vi "from string version 1-0-0.vi"(8 "error in (no error)":errorcluster, 10 "Data String":string, 11 "DAQmx Watchdog configuration in":refnum<class "DAQmx Watchdog configuration.lvclass">) -> (0 "error out":errorcluster, 3 "DAQmx Watchdog configuration out":refnum<class "DAQmx Watchdog configuration.lvclass">)   [LabVIEW 2014, in "DAQmx Watchdog configuration.lvclass"]
uses:
  DAQmx Watchdog configuration.lvclass
  DAQmx Watchdog configuration.lvclass/DAQmx Watchdog configuration.ctl
  <vilib>/NI/Configuration Framework/serializable configuration/NISE_CEF_serializable configuration.lvclass
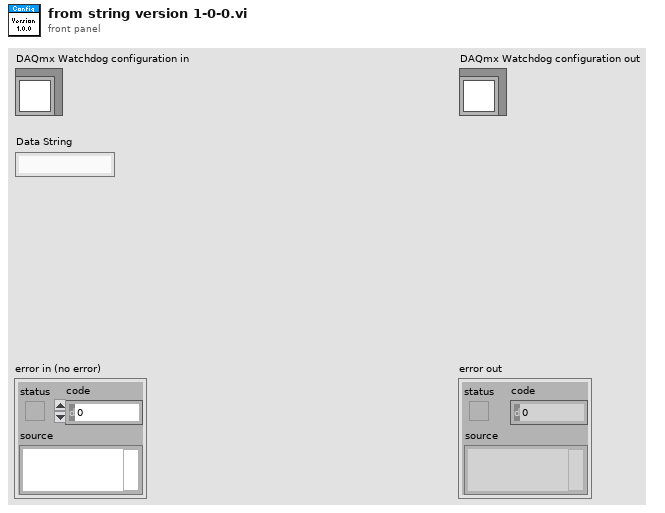
[diagram p1: front panel]
types:
  T1 = cluster{"physical channel(s)":tag, "expiration state":i32}[]
  T2 = cluster{"physical channel":tag, "expiration state":dbl, "output type":i32}[]
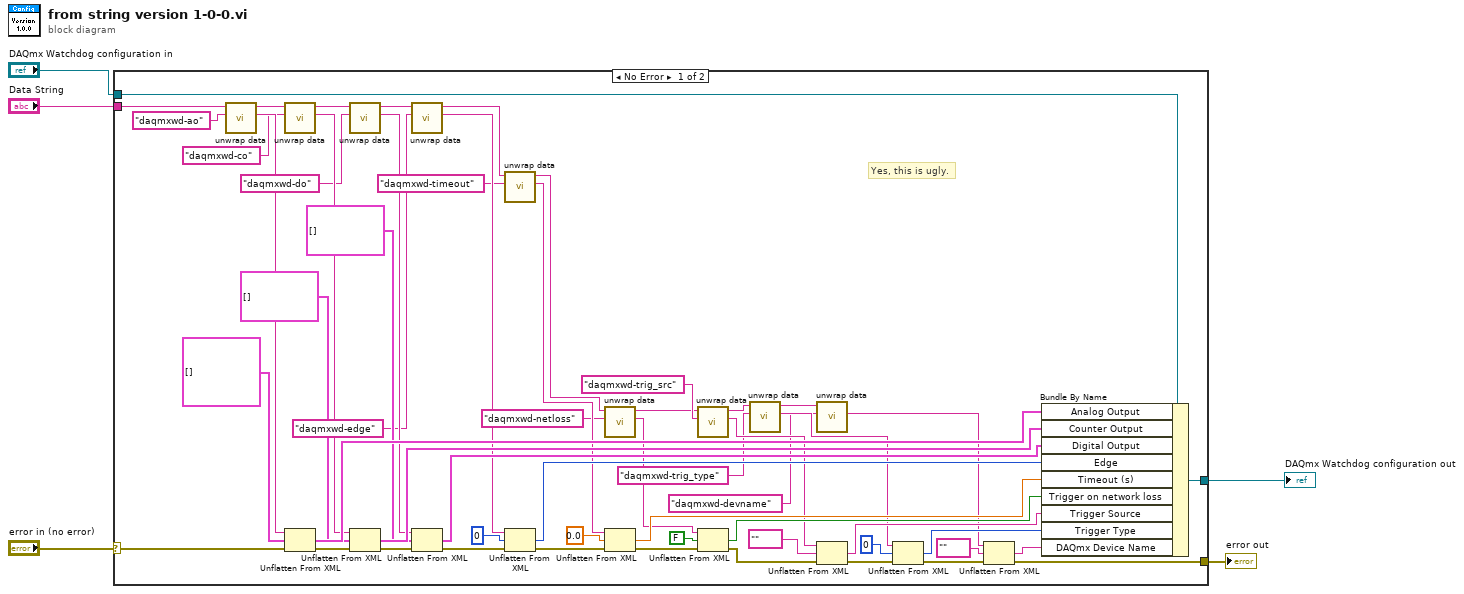
[diagram p0: block diagram]
diagram:
  n1 = case shown="No Error" "error in (no error)" {
    selector: "error in (no error)" -> [w57 w64]
    tunnel: [w7 w64] -> w4
    tunnel: [w61 w63] -> w2
    tunnel: "DAQmx Watchdog configuration in" -> [w62 w63]
    tunnel: "Data String" -> [w55 _]
    frame No Error {
      # "Yes, this is ugly."
      n2 = call <vilib>:"unwrap data.vi"("identifier"="daqmxwd-ao", "data to unwrap"=w55) -> ("unwrapped data"=w59:string, "remaining string"=w53:string)  [unwired: 8 in]
      n3 = call <vilib>:"unwrap data.vi"("identifier"="daqmxwd-co", "data to unwrap"=w53) -> ("unwrapped data"=w52:string, "remaining string"=w47:string)  [unwired: 8 in]
      n4 = Unflatten From XML(xml string=w59, type=T2 [] ("Analog Output"), error in (no error)=w57) -> (value=w56:T2, error out=w49:errorcluster)
      n5 = call <vilib>:"unwrap data.vi"("identifier"="daqmxwd-do", "data to unwrap"=w47) -> ("unwrapped data"=w46:string, "remaining string"=w41:string)  [unwired: 8 in]
      n6 = Unflatten From XML(xml string=w52, type=T1 [] ("Counter Output"), error in (no error)=w49) -> (value=w50:T1, error out=w45:errorcluster)
      n7 = call <vilib>:"unwrap data.vi"("identifier"="daqmxwd-edge", "data to unwrap"=w41) -> ("unwrapped data"=w40:string, "remaining string"=w35:string)  [unwired: 8 in]
      n8 = Unflatten From XML(xml string=w46, type=T1 [] ("Digital Output"), error in (no error)=w45) -> (value=w43:T1, error out=w38:errorcluster)
      n9 = call <vilib>:"unwrap data.vi"("identifier"="daqmxwd-timeout", "data to unwrap"=w35) -> ("unwrapped data"=w32:string, "remaining string"=w29:string)  [unwired: 8 in]
      n10 = Unflatten From XML(xml string=w40, type=0 ("Edge"), error in (no error)=w38) -> (value=w37:i32, error out=w33:errorcluster)
      n11 = call <vilib>:"unwrap data.vi"("identifier"="daqmxwd-netloss", "data to unwrap"=w29) -> ("unwrapped data"=w28:string, "remaining string"=w23:string)  [unwired: 8 in]
      n12 = Unflatten From XML(xml string=w32, type=0.0, error in (no error)=w33) -> (value=w31:dbl, error out=w25:errorcluster)
      n13 = call <vilib>:"unwrap data.vi"("identifier"="daqmxwd-trig_src", "data to unwrap"=w23) -> ("unwrapped data"=w21:string, "remaining string"=w18:string)  [unwired: 8 in]
      n14 = Unflatten From XML(xml string=w28, type=FALSE, error in (no error)=w25) -> (value=w26:bool, error out=w20:errorcluster)
      n15 = call <vilib>:"unwrap data.vi"("identifier"="daqmxwd-trig_type", "data to unwrap"=w18) -> ("unwrapped data"=w15:string, "remaining string"=w11:string)  [unwired: 8 in]
      n16 = call <vilib>:"unwrap data.vi"("identifier"="daqmxwd-devname", "data to unwrap"=w11) -> ("unwrapped data"=w9:string)  [unwired: 8 in, 1 out]
      n17 = Unflatten From XML(xml string=w21, type=tag "" ("Trigger Source"), error in (no error)=w20) -> (value=w19:tag, error out=w14:errorcluster)
      n18 = Unflatten From XML(xml string=w15, type=0 ("Trigger Type"), error in (no error)=w14) -> (value=w13:i32, error out=w8:errorcluster)
      n19 = Unflatten From XML(xml string=w9, type=tag "" ("DAQmx Device Name"), error in (no error)=w8) -> (value=w6:tag, error out=w7:errorcluster)
      n20 = Bundle By Name(cluster=w62, "Analog Output"=w56, "Counter Output"=w50, "Digital Output"=w43, "Edge"=w37, "Timeout (s)"=w31, "Trigger on network loss"=w26, "Trigger Source"=w19, "Trigger Type"=w13, "DAQmx Device Name"=w6) -> (w61:refnum<class "DAQmx Watchdog configuration.lvclass">)
    }
    frame Error {
    }
  }
  "error out" <- w4
  "DAQmx Watchdog configuration out" <- w2
